vi "initparammaker.vi"(11 "GAUSSIAN CLUSTER":T1) -> (3 "initparams":dbl[](array[numeric]))   [LabVIEW 2020]
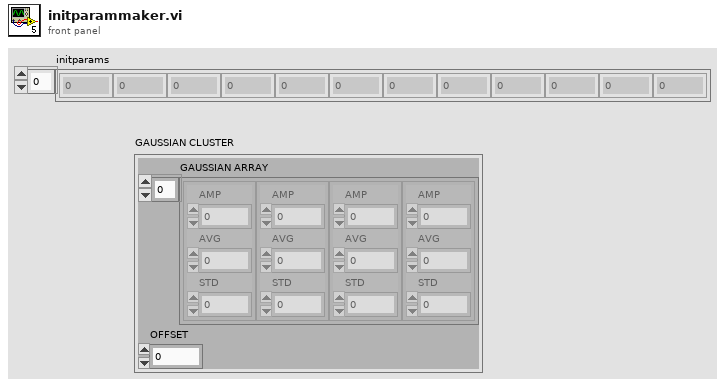
[diagram p1: front panel]
types:
  T1 = cluster{"GAUSSIAN ARRAY":cluster{"AMP":dbl, "AVG":dbl, "STD":dbl}[], "OFFSET":dbl}
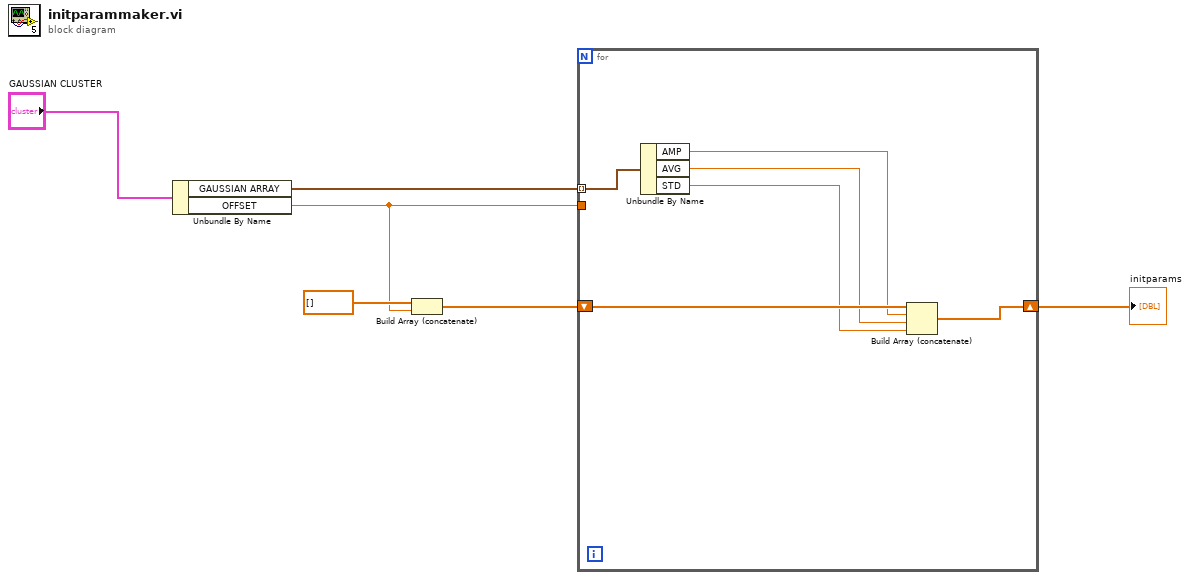
[diagram p0: block diagram]
diagram:
  n1 = Unbundle By Name("GAUSSIAN CLUSTER") -> ("GAUSSIAN ARRAY"=w5:cluster{"AMP":dbl, "AVG":dbl, "STD":dbl}[], "OFFSET"=w3:dbl)
  n2 = Build Array (concatenate)(dbl[] [], w3) -> (w2:dbl[])
  n3 = for {
    tunnel: w5 -> [w12] mode=indexing
    tunnel: w3 -> [_]
    shift-right: [w7] -> w1
    shift-left: w2 -> [w11]
    n4 = Unbundle By Name(w12) -> ("AMP"=w10:dbl, "AVG"=w9:dbl, "STD"=w8:dbl)
    n5 = Build Array (concatenate)(w11, w10, w9, w8) -> (w7:dbl[])
  }
  "initparams" <- w1
